vi "test-cast-speed.vi"() -> ()   [LabVIEW 2019]
uses:
  <vilib>/Rock Robotics/WPI/ThirdParty/JAS_Junk/TrajLib/Trajectory_Library.lvlib
panel:
  out "Total":dbl
  out "Diff":dbl
  out "Numeric":dbl format="%.2f"
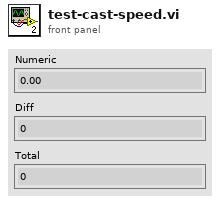
[diagram p1: front panel]
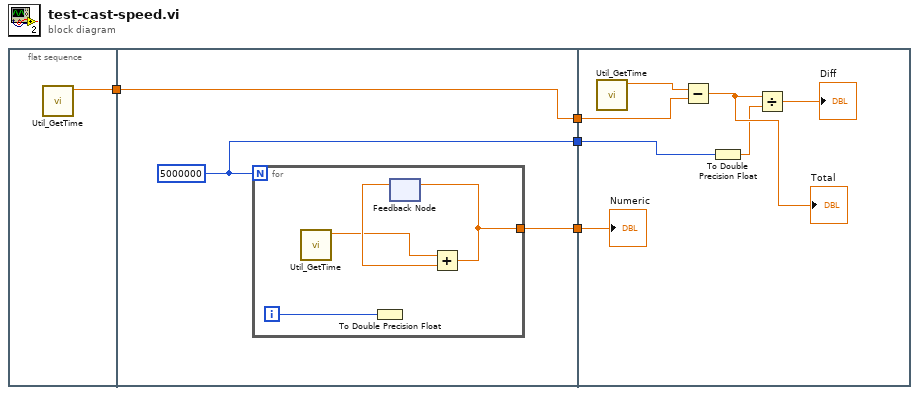
[diagram p0: block diagram]
diagram:
  n1 = flat-sequence {
    tunnel: [w5] -> w4
    tunnel: w4 -> [w8]
    tunnel: [w8] -> w3
    tunnel: [w7] -> w2
    tunnel: [w6] -> w1
    tunnel: w3 -> [w19]
    tunnel: w2 -> [w16]
    tunnel: w1 -> [w13]
    frame #0 {
      n2 = call <vilib>:"Util_GetTime.vi"() -> ("FPGA_Time_Seconds"=w5:dbl)  [unwired: 10 in, 1 out]
    }
    frame #1 {
      w7 = 5000000
      n3 = for {
        N: w7 -> [_]
        tunnel: [w11] -> w6
        i -> [w12]
        n4 = call <vilib>:"Util_GetTime.vi"() -> ("FPGA_Time_Seconds"=w9:dbl)  [unwired: 10 in, 1 out]
        n5 = To Double Precision Float(number=w12) -> ()  [unwired: 1 out]
        n6 = feedback #1() -> (w10:dbl)  [unwired: 1 in]
        n7 = Add(x=w9, y=w10) -> (x+y=w11:dbl)
        n8 = feedback-in #1(w11) -> ()
      }
    }
    frame #2 {
      n9 = call <vilib>:"Util_GetTime.vi"() -> ("FPGA_Time_Seconds"=w14:dbl)  [unwired: 10 in, 1 out]
      n10 = Subtract(x=w14, y=w19) -> (x-y=w17:dbl)
      "Total" <- w17
      n11 = To Double Precision Float(number=w16) -> (double precision float=w15:dbl)
      n12 = Divide(x=w17, y=w15) -> (x/y=→"Diff":dbl)
      "Numeric" <- w13
    }
  }
